vi "Add To Item.vi"(8 "error in":errorcluster, 9 "Item Name":string, 10 "Item node":refnum<k20>, 11 "Parent Item Ref in":refnum<data-value>) -> (0 "error out":errorcluster, 3 "Parent Item Ref out":refnum<data-value>)   [LabVIEW 2024, in "Config File Parser.lvlib"]
uses:
  Config File Parser.lvlib
  Item/Item.lvclass
  <vilib>/xml/Close Reference(Node).vi
  Property/Property.lvclass
  Channel/Channel.lvclass
  Section/Section.lvclass
  <vilib>/xml/NI_XML.lvlib
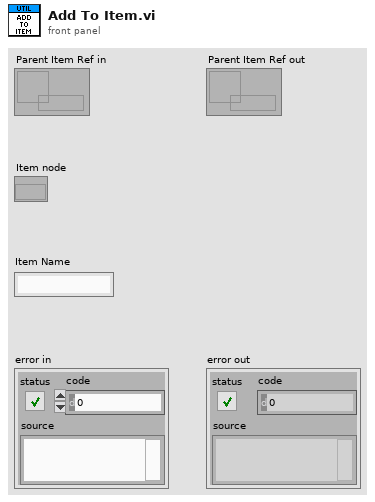
[diagram p1: front panel]
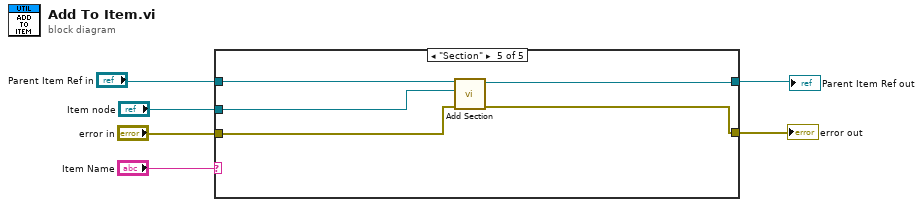
[diagram p0: block diagram]
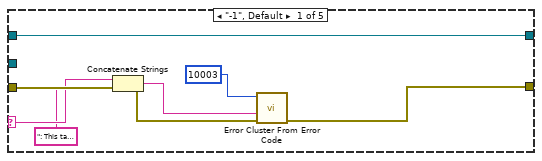
[diagram p2: hidden frame]
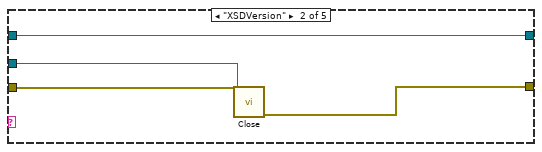
[diagram p3: hidden frame]
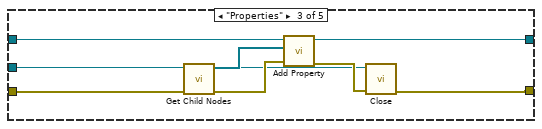
[diagram p4: hidden frame]
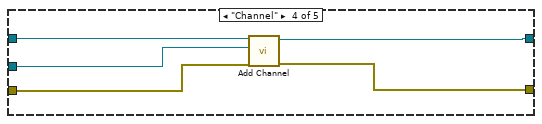
[diagram p5: hidden frame]
diagram:
  n1 = case shown="\"Section\"" "Item Name" {
    selector: "Item Name" -> [w10 _ _ _ _]
    tunnel: "Item node" -> [_ w15 w19 w27 w32]
    tunnel: "Parent Item Ref in" -> [w7 w14 w21 w28 w33]
    tunnel: "error in" -> [w13 w17 w25 w30 w35]
    tunnel: [w12 w16 w23 w29 w34] -> w5
    tunnel: [w7 w14 w18 w26 w31] -> w1
    frame "-1", Default {
      n2 = Concatenate Strings(w10, ": This tag is not allowed. " ("string")) -> (w9:string)
      n3 = call <vilib>:"Error Cluster From Error Code.vi"("error in (no error)"=w13, "error message (\"\")"=w9, "error code (0)"=10003 ("Code")) -> ("error out"=w12:errorcluster)  [unwired: 6 in]
    }
    frame "XSDVersion" {
      n4 = call-poly <vilib>:"Close.vi"("error in (no error)"=w17, "node"=w15) -> ("error out"=w16:errorcluster)  [unwired: 7 in]
    }
    frame "Properties" {
      n5 = call "Get Child Nodes.vi"("error in"=w25, "Node"=w19) -> ("error out"=w24:errorcluster, "Child Nodes"=w20:refnum<k20>[])  [unwired: 8 in]
      n6 = call "Add Property.vi"("error in"=w24, "Property Nodes"=w20, "Item Ref in"=w21) -> ("error out"=w22:errorcluster, "Item Ref out"=w18:refnum<data-value>)  [unwired: 7 in]
      n7 = call-poly <vilib>:"Close.vi"("error in (no error)"=w22, "node"=w19) -> ("error out"=w23:errorcluster)  [unwired: 7 in]
    }
    frame "Channel" {
      n8 = call "Add Channel.vi"("error in"=w30, "Channel Node"=w27, "Item Ref in"=w28) -> ("error out"=w29:errorcluster, "Item Ref out"=w26:refnum<data-value>)  [unwired: 7 in]
    }
    frame "Section" {
      n9 = call "Add Section.vi"("error in"=w35, "Section Node"=w32, "Item Ref in"=w33) -> ("error out"=w34:errorcluster, "Item Ref out"=w31:refnum<data-value>)  [unwired: 7 in]
    }
  }
  "error out" <- w5
  "Parent Item Ref out" <- w1
